vi "Apply params to track.vi"(8 "error in (no error)":errorcluster, 9 "Preserve original timing (T)":bool=TRUE, 10 "Track #":i32=-1) -> (0 "error out":errorcluster)   [LabVIEW 2018, in "Tracks Repair.lvlib"]
doc: "Apply parameters to specific track and save the results.\n_____\nCreated using Delacor QMH Event Scripter 4.2.1.88."
uses:
  Tracks Repair.lvlib
  Apply params to track Argument--cluster.ctl
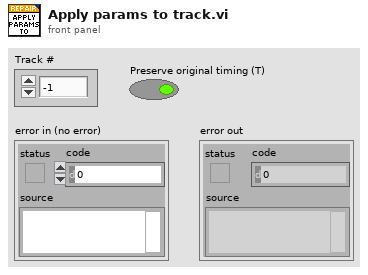
[diagram p1: front panel]
types:
  T1 = typedef "Tracks Repair.lvlib/Apply params to track Argument--cluster.ctl" = cluster{"Track #":i32, "Preserve original timing":bool}
  T2 = typedef "Tracks Repair.lvlib/Request Events--cluster.ctl" = cluster{"Stop Module":refnum<user-event>, "Show Panel":refnum<user-event>, "Hide Panel":refnum<user-event>, "Get Module Execution Status":refnum<user-event>, "Show Diagram":refnum<user-event>, "Open folder":refnum<user-event>, "Load filelist":refnum<user-event>, "Preprocess filelist":refnum<user-event>, "Show list of files":refnum<user-event>, "Load Specific Track":refnum<user-event>, "Show Specific Track":refnum<user-event>, "Process Specific Track":refnum<user-event>, "Update Diagram":refnum<user-event>, "Set Initial View":refnum<user-event>, "Update Settings":refnum<user-event>, "Apply params to track":refnum<user-event>, "Apply to All":refnum<user-event>}
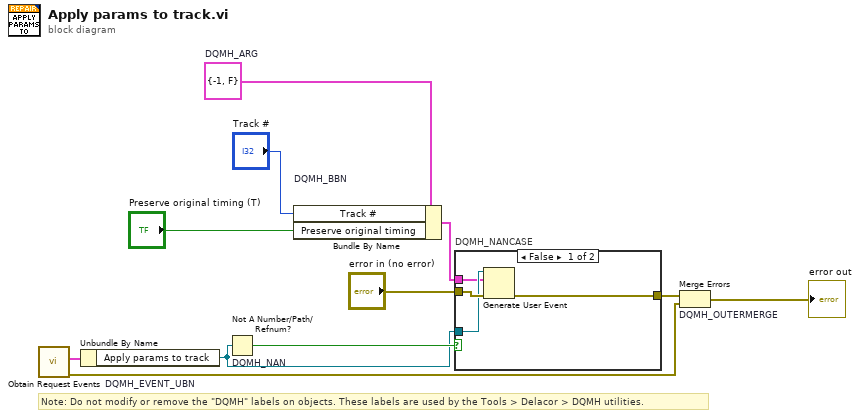
[diagram p0: block diagram]
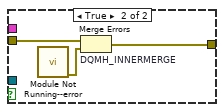
[diagram p2: hidden frame]
diagram:
  w5 = T1 {"Track #"=-1, "Preserve original timing"=FALSE}  # DQMH_ARG
  # "Note: Do not modify or remove the \"DQMH\" labels on objects. These labels are used by the Tools > Delacor > DQMH utilities."
  n1 = call "Obtain Request Events.vi"() -> ("error out"=w3:errorcluster, "Tracks Repair Request Events"=w2:T2)  [unwired: 10 in]
  n2 = Unbundle By Name "DQMH_EVENT_UBN"(w2) -> ("Apply params to track"=w7:refnum<user-event>)
  n3 = Not A Number/Path/Refnum? "DQMH_NAN"(number/path/refnum=w7) -> (NaN/Path/Refnum?=w8:bool)
  n4 = Bundle By Name "DQMH_BBN"(cluster=w5, "Track #"="Track #", "Preserve original timing"="Preserve original timing (T)") -> (w9:T1)
  n5 = case "DQMH_NANCASE" shown="False" w8 {
    tunnel: "error in (no error)" -> [w15 w18]
    tunnel: [w14 w17] -> w6
    tunnel: w7 -> [w13 _]
    tunnel: w9 -> [w12 _]
    frame False {
      n6 = Generate User Event(user event=w13, event data cluster=w12, error in=w15) -> (error out=w14:errorcluster)  [unwired: 1 in, 1 out]
    }
    frame True {
      n7 = call "Module Not Running--error.vi"() -> ("error out"=w16:errorcluster)  [unwired: 11 in]
      n8 = Merge Errors "DQMH_INNERMERGE"(w18, w16) -> (w17:errorcluster)
    }
  }
  n9 = Merge Errors "DQMH_OUTERMERGE"(w6, w3) -> (→"error out":errorcluster)
